vi "Populate Tree.vi"(7 "Indent level":i32, 8 "error in":errorcluster, 9 "Data in":string[](array[string]), 10 "Tags map":refnum<vi>, 11 "TreeControl in":refnum<vi>) -> (0 "error out":errorcluster)   [LabVIEW 2025, in "CAN-LIN Raw Bus Capture UI.lvlib"]
doc: "This VI adds each data row to the tree. Gives back the SIGNALS table data."
uses:
  CAN-LIN Raw Bus Capture UI.lvlib
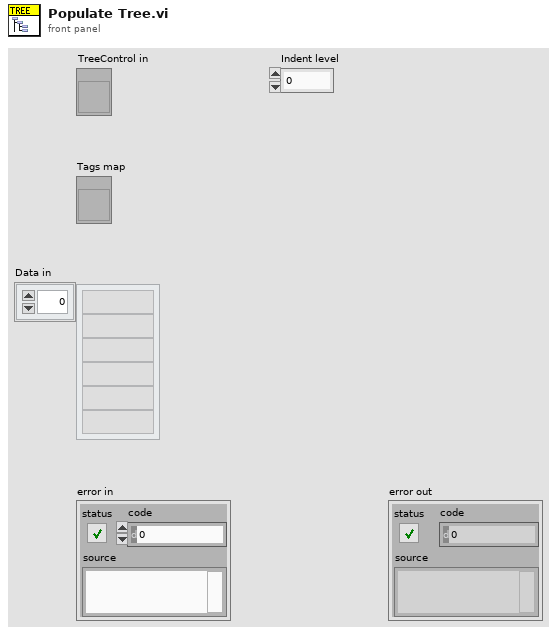
[diagram p1: front panel]
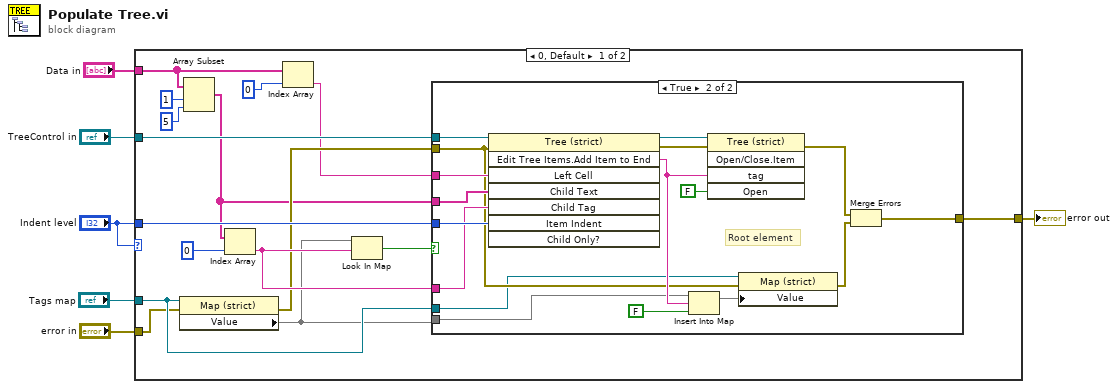
[diagram p0: block diagram]
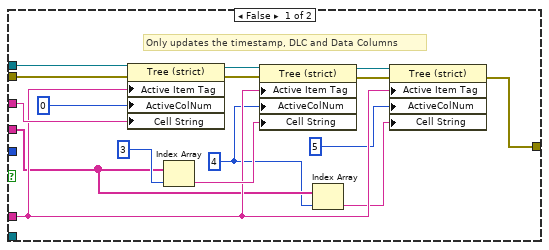
[diagram p2: hidden frame]
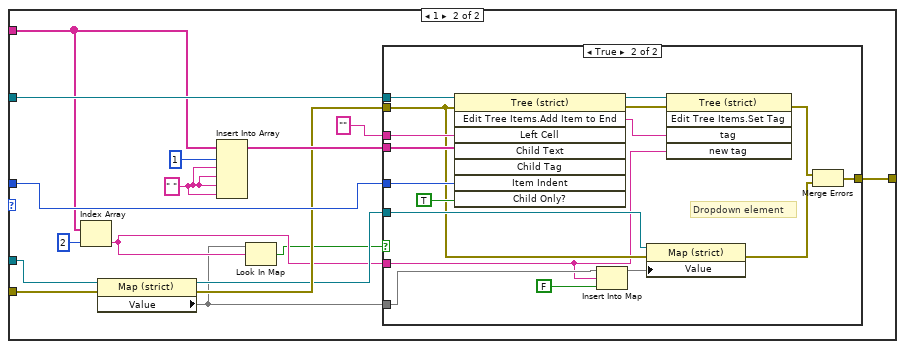
[diagram p3: hidden frame]
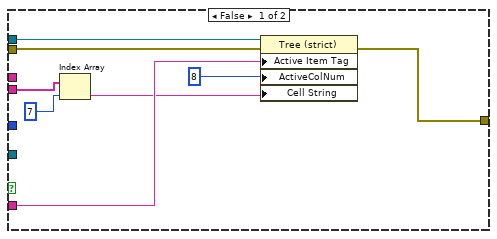
[diagram p4: hidden frame]
diagram:
  n1 = case shown="0, Default" "Indent level" {
    tunnel: "Indent level" -> [w22 w71]
    tunnel: [w21 w70] -> w6
    tunnel: "TreeControl in" -> [w17 w65]
    tunnel: "error in" -> [w16 w63]
    tunnel: "Tags map" -> [w19 w64]
    tunnel: "Data in" -> [w9 w57]
    frame 0, Default {
      n2 = property class="Map (strict)"(reference=w19, error in=w16) -> (error out=w15:errorcluster, "Value"=w13:map{string, bool})  [unwired: 1 out]
      n3 = Array Subset(array=w9, index=1, length=5) -> (w8:string[])
      n4 = Index Array(array=w8, index=0) -> (element=w18:string)
      n5 = Index Array(array=w9, index=0) -> (element=w7:string)
      n6 = Look In Map(map=w13, key=w18) -> (key not found?=w14:bool)  [unwired: 1 in, 1 out]
      n7 = case shown="True" w14 {
        tunnel: w17 -> [w38 w52]
        tunnel: w15 -> [w37 w41]
        tunnel: w22 -> [_ w51]
        tunnel: [w25 w42] -> w21
        tunnel: w7 -> [w35 w50]
        tunnel: w8 -> [w27 w49]
        tunnel: w18 -> [w28 w48]
        tunnel: w19 -> [_ w40]
        tunnel: w13 -> [_ w39]
        frame False {
          w24 = 4 ("index")
          # "Only updates the timestamp, DLC and Data Columns"
          n8 = property class="Tree (strict)"(reference=w38, error in=w37, "Active Item Tag"=w28, "ActiveColNum"=0 ("Active Cell:Active Column Number"), "Cell String"=w35) -> (reference out=w34:refnum<vi>, error out=w33:errorcluster)
          n9 = Index Array(array=w27, index=3 ("Active Cell:Active Column Number")) -> (element=w31:string)
          n10 = property class="Tree (strict)"(reference=w34, error in=w33, "Active Item Tag"=w28, "ActiveColNum"=w24, "Cell String"=w31) -> (reference out=w30:refnum<vi>, error out=w29:errorcluster)
          n11 = Index Array(array=w27, index=w24) -> (element=w26:string)
          n12 = property class="Tree (strict)"(reference=w30, error in=w29, "Active Item Tag"=w28, "ActiveColNum"=5 ("Active Cell:Active Column Number"), "Cell String"=w26) -> (error out=w25:errorcluster)  [unwired: 1 out]
        }
        frame True {
          # "Root element"
          n13 = invoke on="Invoke Node" class="Tree (strict)" method="Edit Tree Items.Add Item to End"(reference=w52, error in=w41, "Left Cell"=w50, "Child Text"=w49, "Child Tag"=w48, "Item Indent"=w51) -> (reference out=w53:refnum<vi>, error out=w55:errorcluster, "Edit Tree Items:Add Item to End"=w47:string)  [unwired: 2 in, 5 out]
          n14 = Insert Into Map(map in=w39, key=w47, value=FALSE) -> (map out=w45:map{string, bool})  [unwired: 2 out]
          n15 = invoke on="Invoke Node" class="Tree (strict)" method="Open/Close.Item"(reference=w53, error in=w55, "tag"=w47, "Open"=FALSE ("Open?")) -> (error out=w44:errorcluster)  [unwired: 1 in, 4 out]
          n16 = property class="Map (strict)"(reference=w40, error in=w41, "Value"=w45) -> (error out=w43:errorcluster)  [unwired: 1 out]
          n17 = Merge Errors(w44, w43) -> (w42:errorcluster)
        }
      }
    }
    frame 1 {
      w67 = " " ("new element/subarray")
      n18 = Index Array(array=w57, index=2) -> (element=w60:string)
      n19 = property class="Map (strict)"(reference=w64, error in=w63) -> (reference out=w61:refnum<vi>, error out=w62:errorcluster, "Value"=w59:map{string, bool})
      n20 = Insert Into Array(array=w57, index=1, new element #1=w67, new element #2=w67, new element #3=w67, new element #4=w67) -> (w68:string[])
      n21 = Look In Map(map=w59, key=w60) -> (key not found?=w58:bool)  [unwired: 1 in, 1 out]
      n22 = case shown="True" w58 {
        tunnel: w71 -> [_ w96]
        tunnel: [w79 w81] -> w70
        tunnel: "" ("Timestamp") -> [_ w95]
        tunnel: w68 -> [w74 w91]
        tunnel: w65 -> [w77 w90]
        tunnel: w60 -> [w78 w80]
        tunnel: w62 -> [w76 w84]
        tunnel: w59 -> [_ w86]
        tunnel: w61 -> [_ w85]
        frame False {
          n23 = Index Array(array=w74, index=7) -> (element=w72:string)
          n24 = property class="Tree (strict)"(reference=w77, error in=w76, "Active Item Tag"=w78, "ActiveColNum"=8 ("Active Cell:Active Column Number"), "Cell String"=w72) -> (error out=w79:errorcluster)  [unwired: 1 out]
        }
        frame True {
          # "Dropdown element"
          n25 = invoke on="Invoke Node" class="Tree (strict)" method="Edit Tree Items.Add Item to End"(reference=w90, error in=w84, "Left Cell"=w95, "Child Text"=w91, "Item Indent"=w96, "Child Only?"=TRUE) -> (reference out=w92:refnum<vi>, error out=w93:errorcluster, "Edit Tree Items:Add Item to End"=w94:string)  [unwired: 2 in, 5 out]
          n26 = Insert Into Map(map in=w86, key=w80, value=FALSE) -> (map out=w87:map{string, bool})  [unwired: 2 out]
          n27 = property class="Map (strict)"(reference=w85, error in=w84, "Value"=w87) -> (error out=w83:errorcluster)  [unwired: 1 out]
          n28 = invoke on="Invoke Node" class="Tree (strict)" method="Edit Tree Items.Set Tag"(reference=w92, error in=w93, "tag"=w94, "new tag"=w80) -> (error out=w82:errorcluster)  [unwired: 1 in, 4 out]
          n29 = Merge Errors(w82, w83) -> (w81:errorcluster)
        }
      }
    }
  }
  "error out" <- w6
